vi "On Script Dialog Opening.vi"(8 "error in (no error)":errorcluster, 10 "Data":T1, 11 "WebView2 Event Filter Interface in":refnum<class "WebView2 Event Filter Interface.lvclass">) -> (0 "error out":errorcluster, 2 "ResultText":string)   [LabVIEW 2025, in "WebView2.lvlib" / "WebView2 Event Filter Interface.lvclass"]
uses:
  WebView2 Event Filter Interface.lvclass
  WebView2 Control Object/Script Dialog Opening Event Data.ctl
  WebView2 Control Object/WebView2 Control.lvclass
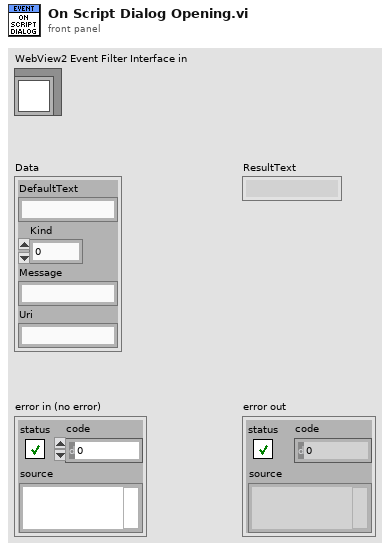
[diagram p1: front panel]
types:
  T1 = typedef "WebView2.lvlib/WebView2 Control.lvclass/Script Dialog Opening Event Data.ctl" = cluster{"DefaultText":string, "Kind":i32, "Message":string, "Uri":string}
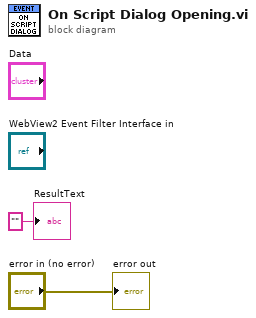
[diagram p0: block diagram]
diagram:
  "error out" <- "error in (no error)"
  "ResultText" <- "" ("ResultText")
